vi "Plane Fit.vi"(7 "Reset Button":bool, 8 "Rough Adjust":dbl, 9 "Fine Adjust":dbl=3.5, 10 "Nano Z":dbl, 11 "Positions":T1 {"z (mm)" format="%.1p"; "y (nm)" format="%.1p"; "x (nm)" format="%.1p"}) -> (2 "Output":dbl, 3 "Clicks":dbl)   [LabVIEW 2017]
uses:
  Program Files/National Instruments/LabVIEW 2019/user.lib/HapticSTM/HapticSTM.lvlib
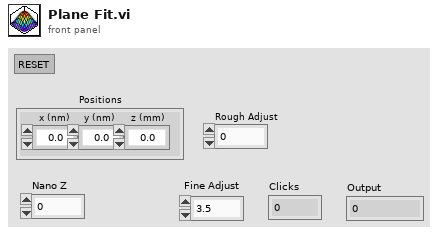
[diagram p1: front panel]
types:
  T1 = cluster{"x (nm)":dbl, "y (nm)":dbl, "z (mm)":dbl}
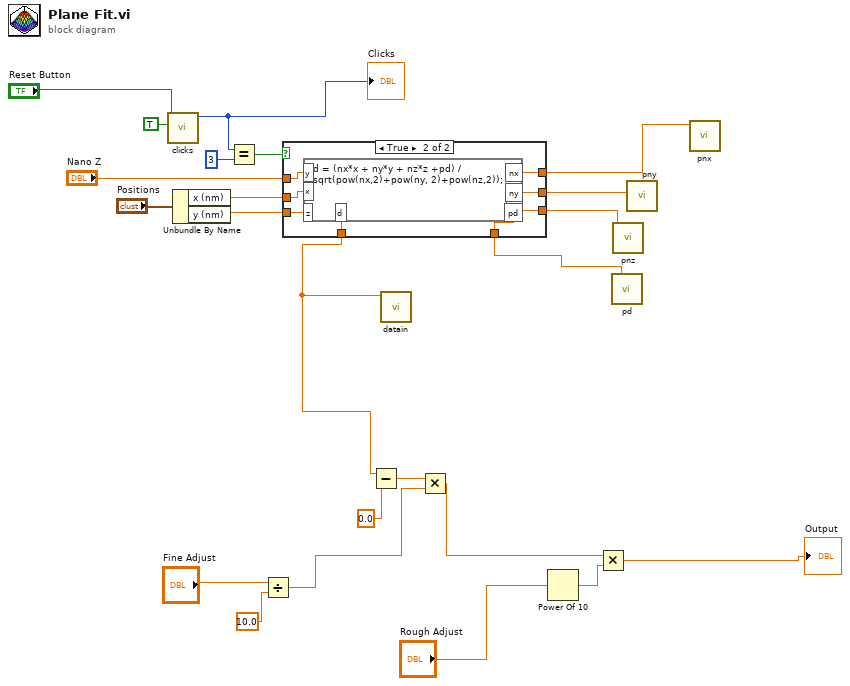
[diagram p0: block diagram]
diagram:
  n1 = call "clicks.vi"("planing"=TRUE, "reset"="Reset Button") -> ("function return"=w16:i32)  [unwired: 9 in]
  "Clicks" <- w16
  n2 = Unbundle By Name("Positions") -> ("x (nm)"=w7:dbl, "y (nm)"=w6:dbl)
  n3 = Equal?(x=w16, y=3) -> (x = y?=w14:bool)
  n4 = Divide(x="Fine Adjust", y=10.0) -> (x/y=w22:dbl)
  n5 = Power Of 10(x="Rough Adjust") -> (10^x=w5:dbl)
  n6 = call "pd.vi"() -> ("function return"=w17:dbl)  [unwired: 11 in]
  n7 = call "pnz.vi"() -> ("function return"=w18:dbl)  [unwired: 11 in]
  n8 = call "pny.vi"() -> ("function return"=w12:dbl)  [unwired: 11 in]
  n9 = call "pnx.vi"() -> ("function return"=w13:dbl)  [unwired: 11 in]
  n10 = case shown="True" w14 {
    tunnel: [w24 w32] -> w10
    tunnel: w13 -> [_ w31]
    tunnel: w12 -> [_ w30]
    tunnel: w18 -> [_ w29]
    tunnel: w17 -> [_ w28]
    tunnel: "Nano Z" -> [w24 w27]
    tunnel: w7 -> [_ w26]
    tunnel: w6 -> [_ w25]
    frame False {
    }
    frame True {
      n11 = formula code="d = (nx*x + ny*y + nz*z +pd) / sqrt(pow(nx,2)+pow(ny, 2)+pow(nz,2));"("y"=w27, "z"=w25, "x"=w26, "nx"=w31, "ny"=w30, "nz"=w29, "pd"=w28) -> ("d"=w32:dbl)
    }
  }
  n12 = Subtract(x=w10, y=0.0 ("x")) -> (x-y=w23:dbl)
  n13 = call "datain.vi"("output"=w10) -> ()  [unwired: 11 in]
  n14 = Multiply(x=w23, y=w22) -> (x*y=w3:dbl)
  n15 = Multiply(x=w3, y=w5) -> (x*y=→"Output":dbl)
